vi "Sub_Report_Generation.vi"(8 "error in (no error)":errorcluster caption="에러 입력(에러 없음)", 11 "File Name":string) -> (0 "error out":errorcluster caption="에러 출력", 2 "cal fac B":dbl format="%.2f", 3 "cal fac A":dbl format="%.2f")   [LabVIEW 2015]
uses:
  <vilib>/addons/_office/excel.llb/Excel Easy Table (num).vi
  <vilib>/addons/_office/excel.llb/Excel Get Data (dbl).vi
  <vilib>/Utility/NIReport.llb/NI_report.lvclass
  <vilib>/addons/_office/NI_ReportGenerationToolkit.lvlib
  <vilib>/Utility/NIReport.llb/Excel/NI_Excel.lvclass
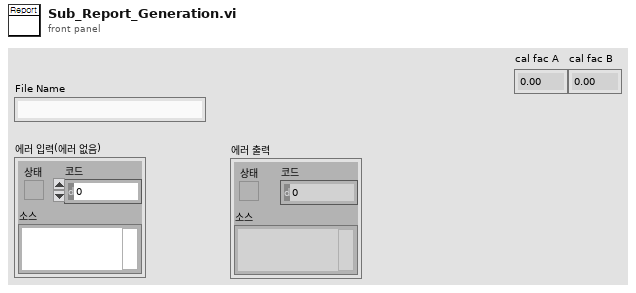
[diagram p1: front panel]
types:
  T1 = enum16{"Standard Report", "HTML", "Word", "Excel"}
  T2 = enum16{"maximized", "minimized", "normal", "no change"}
  T3 = cluster{"Load":dbl[], "LWA":dbl[], "LWB":dbl[], "LWC":dbl[], "RWA":dbl[], "RWB":dbl[], "RWC":dbl[], "Bat":u16[]}
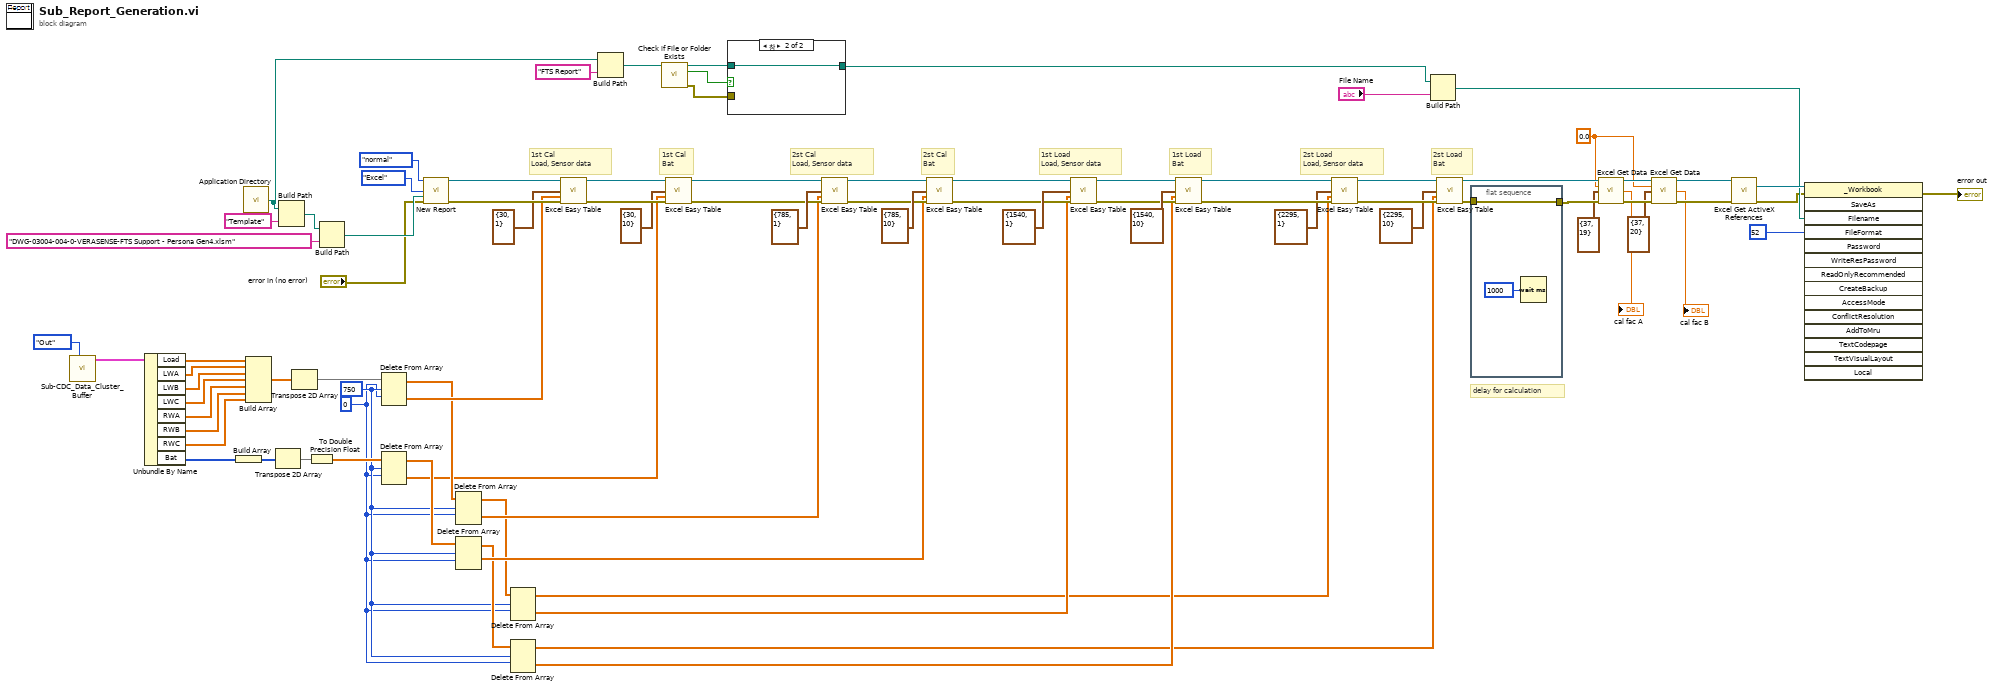
[diagram p0: block diagram]
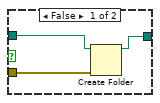
[diagram p2: hidden frame]
diagram:
  w7 = 0.0
  w31 = 0 ("인덱스 (행)")
  w32 = 750 ("길이")
  # "delay for calculation"
  # "2st Load\nBat"
  # "2st Load\nLoad, Sensor data"
  # "1st Load\nBat"
  # "1st Load\nLoad, Sensor data"
  # "2st Cal\nBat"
  # "2st Cal\nLoad, Sensor data"
  # "1st Cal\nBat"
  # "1st Cal\nLoad, Sensor data"
  n1 = call "Sub-CDC_Data_Cluster_Buffer.vi"("Mode"=enum16{"Init", "Add", "Add Load", "Out"}."Out") -> ("Output CL"=w76:T3)  [unwired: 10 in]
  n2 = Unbundle By Name(w76) -> ("Load"=w75:dbl[], "LWA"=w74:dbl[], "LWB"=w73:dbl[], "LWC"=w72:dbl[], "RWA"=w71:dbl[], "RWB"=w70:dbl[], "RWC"=w69:dbl[], "Bat"=w50:u16[])
  n3 = Build Array(w50) -> (w61:u16[][])
  n4 = call <vilib>:"Application Directory.vi"() -> ("Application Directory"=w26:path)
  n5 = Build Array(w75, w74, w73, w72, w71, w70, w69) -> (w68:dbl[][])
  n6 = Transpose 2D Array(2D array=w61) -> (transposed array=w60:u16[][])
  n7 = Build Path(base path=w26, name or relative path="Template" ("이름 또는 상대 경로")) -> (appended path=w82:path)
  n8 = Transpose 2D Array(2D array=w68) -> (transposed array=w67:dbl[][])
  n9 = To Double Precision Float(number=w60) -> (double precision float=w49:dbl[][])
  n10 = Build Path(base path=w82, name or relative path="DWG-03004-004-0-VERASENSE-FTS Support - Persona Gen4.xlsm" ("이름 또는 상대 경로")) -> (appended path=w80:path)
  n11 = Delete From Array(array=w67, length=w32, index (row)=w31) -> (deleted portion=w66:dbl[][], array with subset deleted=w59:dbl[][])  [unwired: 1 in]
  n12 = Delete From Array(array=w49, length=w32, index (row)=w31) -> (deleted portion=w47:dbl[][], array with subset deleted=w58:dbl[][])  [unwired: 1 in]
  n13 = call <vilib>:"New Report.vi"("window state (normal)"=T2."normal", "report type"=T1."Excel", "template (empty)"=w80, "error in (no error)"="error in (no error)") -> ("report out"=w79:refnum<class "NI_report.lvclass">, "error out"=w78:errorcluster)  [unwired: 10 in]
  n14 = Delete From Array(array=w59, length=w32, index (row)=w31) -> (deleted portion=w51:dbl[][], array with subset deleted=w34:dbl[][])  [unwired: 1 in]
  n15 = Delete From Array(array=w58, length=w32, index (row)=w31) -> (deleted portion=w48:dbl[][], array with subset deleted=w33:dbl[][])  [unwired: 1 in]
  n16 = Delete From Array(array=w34, length=w32, index (row)=w31) -> (deleted portion=w30:dbl[][], array with subset deleted=w28:dbl[][])  [unwired: 1 in]
  n17 = Delete From Array(array=w33, length=w32, index (row)=w31) -> (deleted portion=w29:dbl[][], array with subset deleted=w27:dbl[][])  [unwired: 1 in]
  n18 = call-poly <vilib>:"Excel Easy Table.vi"("report in"=w79, "start (0, 0)"=cluster{"row":i32, "column":i32} {"row"=30, "column"=1}, "text data"=w66, "error in (no error)"=w78) -> ("report out"=w64:refnum<class "NI_report.lvclass">, "error out"=w63:errorcluster)  [unwired: 7 in, 3 out]
  n19 = Build Path(base path=w26, name or relative path="FTS Report" ("이름 또는 상대 경로")) -> (appended path=w21:path)
  n20 = call <vilib>:"Check if File or Folder Exists.vi"("path"=w21) -> ("error out"=w22:errorcluster, "file or folder exists?"=w24:bool, "dup path"=w23:path)  [unwired: 8 in]
  n21 = call-poly <vilib>:"Excel Easy Table.vi"("report in"=w64, "start (0, 0)"=cluster{"row":i32, "column":i32} {"row"=30, "column"=10}, "text data"=w47, "error in (no error)"=w63) -> ("report out"=w53:refnum<class "NI_report.lvclass">, "error out"=w52:errorcluster)  [unwired: 7 in, 3 out]
  n22 = case shown="참" w24 {
    tunnel: w23 -> [w88 w89]
    tunnel: w22 -> [w87 _]
    tunnel: [w86 w89] -> w20
    frame False {
      n23 = Create Folder(path (use dialog)=w88, error in=w87) -> (created path=w86:path)  [unwired: 1 in, 2 out]
    }
    frame True {
    }
  }
  n24 = call-poly <vilib>:"Excel Easy Table.vi"("report in"=w53, "start (0, 0)"=cluster{"row":i32, "column":i32} {"row"=785, "column"=1}, "text data"=w51, "error in (no error)"=w52) -> ("report out"=w55:refnum<class "NI_report.lvclass">, "error out"=w56:errorcluster)  [unwired: 7 in, 3 out]
  n25 = call-poly <vilib>:"Excel Easy Table.vi"("report in"=w55, "start (0, 0)"=cluster{"row":i32, "column":i32} {"row"=785, "column"=10}, "text data"=w48, "error in (no error)"=w56) -> ("report out"=w36:refnum<class "NI_report.lvclass">, "error out"=w35:errorcluster)  [unwired: 7 in, 3 out]
  n26 = call-poly <vilib>:"Excel Easy Table.vi"("report in"=w36, "start (0, 0)"=cluster{"row":i32, "column":i32} {"row"=1540, "column"=1}, "text data"=w30, "error in (no error)"=w35) -> ("report out"=w38:refnum<class "NI_report.lvclass">, "error out"=w39:errorcluster)  [unwired: 7 in, 3 out]
  n27 = call-poly <vilib>:"Excel Easy Table.vi"("report in"=w38, "start (0, 0)"=cluster{"row":i32, "column":i32} {"row"=1540, "column"=10}, "text data"=w29, "error in (no error)"=w39) -> ("report out"=w45:refnum<class "NI_report.lvclass">, "error out"=w46:errorcluster)  [unwired: 7 in, 3 out]
  n28 = call-poly <vilib>:"Excel Easy Table.vi"("report in"=w45, "start (0, 0)"=cluster{"row":i32, "column":i32} {"row"=2295, "column"=1}, "text data"=w28, "error in (no error)"=w46) -> ("report out"=w43:refnum<class "NI_report.lvclass">, "error out"=w42:errorcluster)  [unwired: 7 in, 3 out]
  n29 = Build Path(base path=w20, name or relative path="File Name") -> (appended path=w15:path)
  n30 = call-poly <vilib>:"Excel Easy Table.vi"("report in"=w43, "start (0, 0)"=cluster{"row":i32, "column":i32} {"row"=2295, "column"=10}, "text data"=w27, "error in (no error)"=w42) -> ("report out"=w13:refnum<class "NI_report.lvclass">, "error out"=w12:errorcluster)  [unwired: 7 in, 3 out]
  n31 = flat-sequence {
    tunnel: w12 -> [w91]
    tunnel: [w91] -> w11
    frame #0 {
      n32 = Wait (ms)(milliseconds to wait=u32 1000 ("대기 시간(ms)")) -> ()  [unwired: 1 out]
    }
  }
  n33 = call-poly <vilib>:"Excel Get Data.vi"("report in"=w13, "data type"=w7, "start (0, 0)"=cluster{"start row":i32, "start column":i32} {"start row"=37, "start column"=19}, "error in (no error)"=w11) -> ("report out"=w9:refnum<class "NI_report.lvclass">, "data"=→"cal fac A":dbl, "error out"=w8:errorcluster)  [unwired: 9 in]
  n34 = call-poly <vilib>:"Excel Get Data.vi"("report in"=w9, "data type"=w7, "start (0, 0)"=cluster{"start row":i32, "start column":i32} {"start row"=37, "start column"=20}, "error in (no error)"=w8) -> ("report out"=w5:refnum<class "NI_report.lvclass">, "data"=→"cal fac B":dbl, "error out"=w4:errorcluster)  [unwired: 9 in]
  n35 = call <vilib>:"Excel Get ActiveX References.vi"("report in"=w5, "error in (no error)"=w4) -> ("Excel._Workbook"=w17:refnum<k7>, "error out"=w1:errorcluster)  [unwired: 7 in, 5 out]
  n36 = invoke on="인보크 노드" class="_Workbook" method="SaveAs"(reference=w17, error in=w1, "Filename"=w15, "FileFormat"=52) -> (error out=→"error out":errorcluster)  [unwired: 11 in, 14 out]
